vi "LCR_TrimOC.vi"(8 "error in (no error)":errorcluster, 11 "LCRControl in":refnum<class "LCRControl.lvclass">) -> (0 "error out":errorcluster, 3 "LCRControl out":refnum<class "LCRControl.lvclass">)   [LabVIEW 2013, in "LCRControl.lvclass"]
uses:
  LCRControl.lvclass
  InstrControl.lvclass
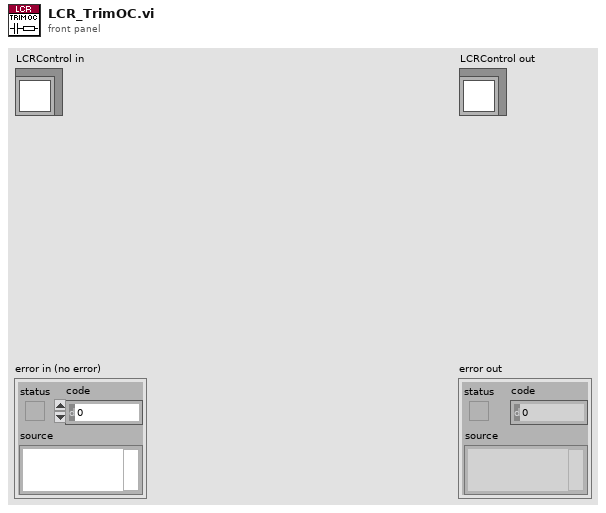
[diagram p1: front panel]
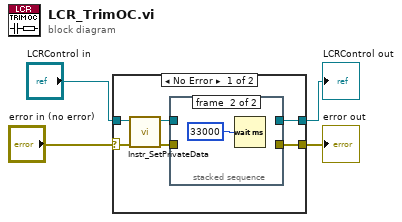
[diagram p0: block diagram]
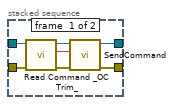
[diagram p2: hidden frame]
diagram:
  n1 = case shown="No Error" "error in (no error)" {
    selector: "error in (no error)" -> [w7 w20]
    tunnel: [w9 w20] -> w3
    tunnel: [w10 w19] -> w1
    tunnel: "LCRControl in" -> [w8 w19]
    frame No Error {
      n2 = call-dynamic "Instr_SetPrivateData.vi"("error in (no error)"=w7, "LCRControl in"=w8) -> ("error out"=w6:errorcluster, "LCRControl out"=w5:refnum<class "LCRControl.lvclass">)  [unwired: 8 in]
      n3 = stacked-sequence {
        tunnel: [w17 _] -> w10
        tunnel: w6 -> [w13 _]
        tunnel: [w12 _] -> w9
        tunnel: w5 -> [w11 _]
        frame #0 {
          n4 = call-dynamic "Read Command _OC Trim_.vi"("error in (no error)"=w13, "LCRControl in"=w11) -> ("error out"=w14:errorcluster, "Command \"OC Trim\""=w15:string, "LCRControl out"=w16:refnum<class "LCRControl.lvclass">)  [unwired: 7 in]
          n5 = call "SendCommand.vi"("error in (no error)"=w14, "Command string"=w15, "InstControl in"=w16) -> ("error out"=w12:errorcluster, "InstControl out"=w17:refnum<class "LCRControl.lvclass">)  [unwired: 7 in]
        }
        frame #1 {
          n6 = Wait (ms)(milliseconds to wait=33000) -> ()  [unwired: 1 out]
        }
      }
    }
    frame Error {
    }
  }
  "error out" <- w3
  "LCRControl out" <- w1
